vi "Shooter Suggestion.vi"(6 "Distance":dbl, 9 "Suggest":bool, 10 "Radius in":dbl[](array[numeric]), 11 "Theta in":dbl[](array[numeric])) -> (2 "Radius out":dbl[](array[numeric]), 3 "Theta Out":dbl[](array[numeric]))   [LabVIEW 2011]
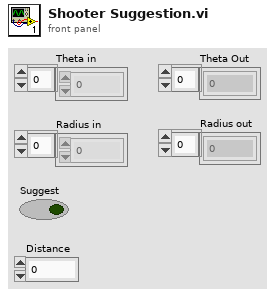
[diagram p1: front panel]
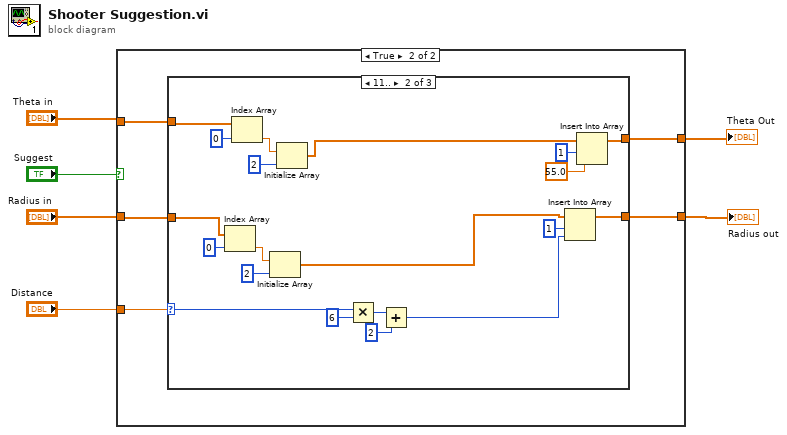
[diagram p0: block diagram]
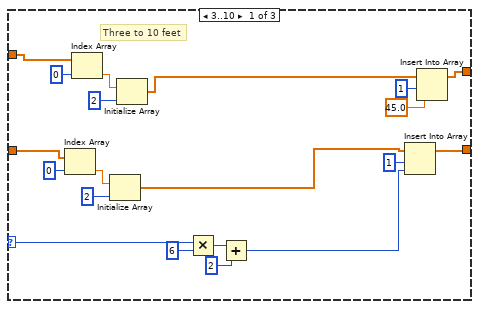
[diagram p3: hidden frame]
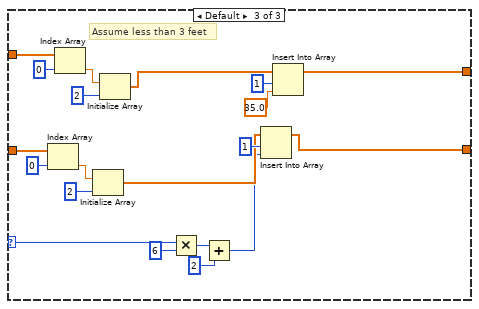
[diagram p4: hidden frame]
diagram:
  n1 = case shown="True" "Suggest" {
    tunnel: "Theta in" -> [w8 w12]
    tunnel: [w8 w11] -> w3
    tunnel: "Radius in" -> [w7 w10]
    tunnel: [w7 w9] -> w5
    tunnel: "Distance" -> [_ w13]
    frame False {
    }
    frame True {
      n2 = case shown="11.." w13 {
        selector: w13 -> [w15 w36 w59]
        tunnel: w12 -> [w18 w38 w72]
        tunnel: [w17 w34 w66] -> w11
        tunnel: w10 -> [w14 w37 w62]
        tunnel: [w16 w35 w54] -> w9
        frame 3..10 {
          # "Three to 10 feet"
          n3 = Index Array(array=w14, index=0) -> (element=w26:dbl)
          n4 = Index Array(array=w18, index=0) -> (element=w20:dbl)
          n5 = Initialize Array(w26, 2 ("dimension size")) -> (w29:dbl[])
          n6 = Initialize Array(w20, 2 ("dimension size")) -> (w22:dbl[])
          n7 = Multiply(x=w15, y=6) -> (x*y=w31:i32)
          n8 = Add(x=w31, y=2) -> (x+y=w33:i32)
          n9 = Insert Into Array(array=w29, index=1, new element=w33) -> (w16:dbl[])
          n10 = Insert Into Array(array=w22, index=1, new element=45.0 ("new element/subarray")) -> (w17:dbl[])
        }
        frame 11.. {
          n11 = Index Array(array=w37, index=0) -> (element=w46:dbl)
          n12 = Index Array(array=w38, index=0) -> (element=w40:dbl)
          n13 = Initialize Array(w46, 2 ("dimension size")) -> (w49:dbl[])
          n14 = Initialize Array(w40, 2 ("dimension size")) -> (w42:dbl[])
          n15 = Multiply(x=w36, y=6) -> (x*y=w51:i32)
          n16 = Add(x=w51, y=2) -> (x+y=w53:i32)
          n17 = Insert Into Array(array=w49, index=1, new element=w53) -> (w35:dbl[])
          n18 = Insert Into Array(array=w42, index=1, new element=55.0 ("new element/subarray")) -> (w34:dbl[])
        }
        frame Default {
          # "Assume less than 3 feet"
          n19 = Index Array(array=w62, index=0) -> (element=w64:dbl)
          n20 = Index Array(array=w72, index=0) -> (element=w71:dbl)
          n21 = Initialize Array(w64, 2 ("dimension size")) -> (w60:dbl[])
          n22 = Initialize Array(w71, 2 ("dimension size")) -> (w69:dbl[])
          n23 = Multiply(x=w59, y=6) -> (x*y=w57:i32)
          n24 = Add(x=w57, y=2) -> (x+y=w55:i32)
          n25 = Insert Into Array(array=w60, index=1, new element=w55) -> (w54:dbl[])
          n26 = Insert Into Array(array=w69, index=1, new element=35.0 ("new element/subarray")) -> (w66:dbl[])
        }
      }
    }
  }
  "Radius out" <- w5
  "Theta Out" <- w3
